vi "openCoGFile.vi"(8 "error in (no error)":errorcluster, 10 "nbrCol":i32, 11 "Logging Configuration":T1 {"NbrIma" min=1 step=1}) -> (0 "error out":errorcluster)   [LabVIEW 2020]
uses:
  LOGGING/Logging Configuration.ctl
  DataTyp_Header.ctl
  ClustBigFilFits.ctl
  BigDataFits.ctl
  LOGGING/Logging.lvlib
panel:
  in  "name":string="centerofgravity"
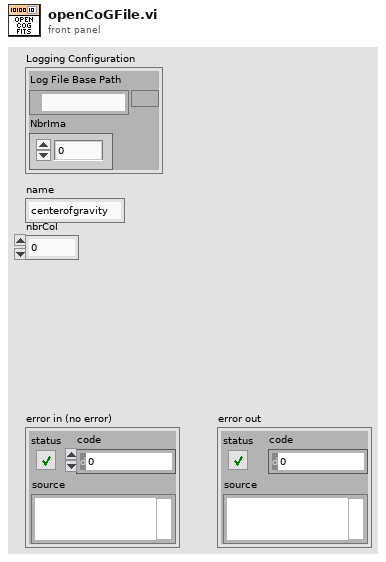
[diagram p1: front panel]
types:
  T1 = typedef "Logging.lvlib/Logging Configuration.ctl" = cluster{"Log File Base Path":path, "NbrIma":i32}
  T2 = typedef "BigDataFits.ctl" = enum16{"Init", "WritHeader", "WritData", "Close"}
  T3 = typedef "ClustBigFilFits.ctl" = cluster{"file (use dialog)":path, "Type de données":T4, "Commentaire":string, "naxis1":i32, "naxis2":i32, "naxis3":i32, "Exptime":sgl}
  T4 = typedef "DataTyp_Header.ctl" = enum16{"U8 (unsigned integer 8bit)", "I16 (signed integer 16bit)", "U16 (unsigned integer 16 bit)", "I32 (signed integer 32bit)", "U32 (unsigned integer 32 bit)", "SGL (float 32bit)", "DBL(float 64bit)", "complex (2xfloat 64bit)"}
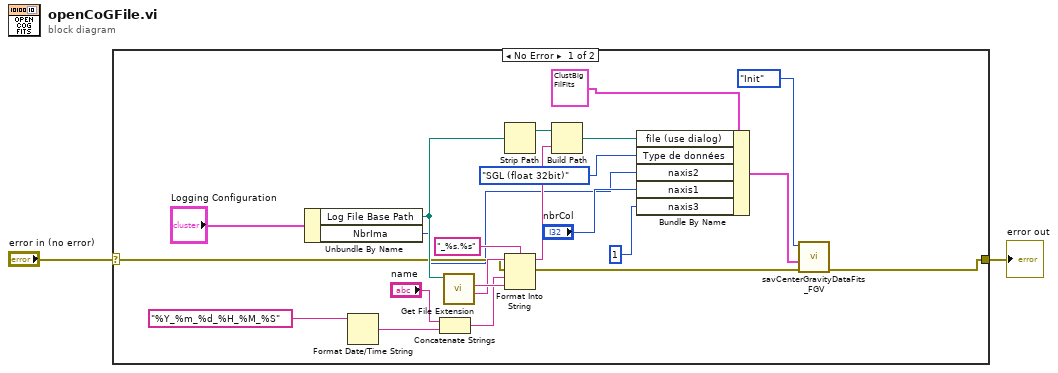
[diagram p0: block diagram]
diagram:
  n1 = case shown="No Error" "error in (no error)" {
    selector: "error in (no error)" -> [w10 w25]
    tunnel: [w6 w25] -> w2
    frame No Error {
      n2 = Unbundle By Name("Logging Configuration") -> ("Log File Base Path"=w13:path, "NbrIma"=w3:i32)
      n3 = Format Date/Time String(time format string (%c)="%Y_%m_%d_%H_%M_%S") -> (date/time string=w18:string)  [unwired: 2 in]
      n4 = Concatenate Strings("name", w18) -> (w12:string)
      n5 = call <vilib>:"Get File Extension.vi"("file"=w13) -> ("filename without extension"=w15:string, "lowercase file extension"=w19:string)  [unwired: 6 in, 3 out]
      n6 = Strip Path(path=w13) -> (stripped path=w16:path)  [unwired: 1 out]
      n7 = Format Into String(format string="_%s.%s", initial string=w15, error in=w10, w12, w19) -> (resulting string=w20:string, error out=w8:errorcluster)
      n8 = Build Path(base path=w16, name or relative path=w20) -> (appended path=w23:path)
      n9 = Bundle By Name(cluster=T3 {"file (use dialog)"=path "D:/DATA/Imatest.fits", "Type de données"=enum."U16 (unsigned integer 16 bit)", "Commentaire"="", "naxis1"=0, "naxis2"=0, "naxis3"=1, "Exptime"=1.0} ("ClustBigFilFits"), "file (use dialog)"=w23, "Type de données"=DataTyp_Header."SGL (float 32bit)", "naxis2"=w3, "naxis1"="nbrCol", "naxis3"=1) -> (w7:T3)
      n10 = call "savCenterGravityDataFits_FGV.vi"("InError"=w8, "Cluster"=w7, "Énum"=BigDataFits."Init") -> ("sortie d'erreur"=w6:errorcluster)  [unwired: 8 in]
    }
    frame Error {
    }
  }
  "error out" <- w2
